vi "Error-Format Stack.vi"() -> (8 "formatted stack":string)   [LabVIEW 2020]
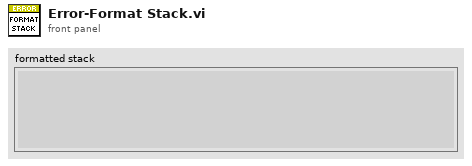
[diagram p1: front panel]
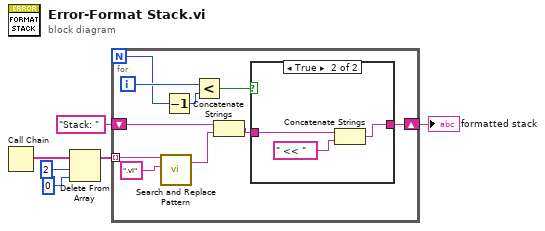
[diagram p0: block diagram]
diagram:
  n1 = Call Chain() -> (call chain=w3:string[])
  n2 = Delete From Array(array=w3, length=2, index=0) -> (array with subset deleted=w6:string[])  [unwired: 1 out]
  n3 = for {
    N -> [w10]
    tunnel: w6 -> [w16] mode=indexing
    shift-right: [w7] -> w1
    shift-left: "Stack: " -> [w14]
    i -> [w12]
    n4 = call <vilib>:"Search and Replace Pattern.vi"("string"=w16, "regular expression (\"\")"=".vi") -> ("result string"=w13:string)  [unwired: 3 in, 1 out]
    n5 = Decrement(x=w10) -> (x-1=w11:i32)
    n6 = Less?(x=w12, y=w11) -> (x < y?=w9:bool)
    n7 = Concatenate Strings(w14, w13) -> (w8:string)
    n8 = case shown="True" w9 {
      tunnel: w8 -> [w17 w20]
      tunnel: [w17 w19] -> w7
      frame False {
      }
      frame True {
        n9 = Concatenate Strings(w20, " << " ("string")) -> (w19:string)
      }
    }
  }
  "formatted stack" <- w1
